vi "Command Information--SubVI.vi"(8 "error in (no error)":errorcluster, 9 "Instance":i32=1, 10 "Commands":T1=enum."Temp Feedback", 11 "Watlow F4T In":refnum<class "Watlow F4T.lvclass">) -> (0 "error out":errorcluster, 1 "Found?":bool, 2 "Register":T2, 3 "Watlow F4T Out":refnum<class "Watlow F4T.lvclass">)   [LabVIEW 2024, in "Watlow F4T.lvclass"]
uses:
  Watlow F4T.lvclass
  Controls/Standard Bus Register LUT Data--Cluster.ctl
  Controls/Standard Bus Commands--Enum.ctl
  Controls/Standard Bus Class Names--Enum.ctl
  Controls/Standard Bus Parameter Names--Enum.ctl
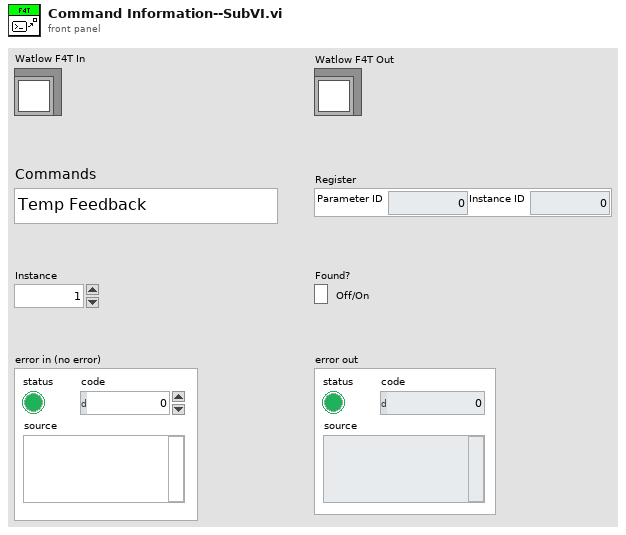
[diagram p1: front panel]
types:
  T1 = typedef "Watlow F4T.lvclass/Standard Bus Commands--Enum.ctl" = enum16{"Remote Setpoint", "Remote Mode", "Temp Feedback", "Target Setpoint", "Current Setpoint", "Setpoint Lower Limit", "Setpoint Upper Limit", "Ramp Rate Y", "Ramp Rate X", "Ramp Rate Action", "Temp Control State", "Temp Control Mode", "Power", "Heat Power", "Cool Power"}
  T2 = typedef "Watlow F4T.lvclass/Standard Bus Register LUT Data--Cluster.ctl" = cluster{"Parameter ID":i32, "Instance ID":i32}
  T3 = typedef "Watlow F4T.lvclass/Standard Bus Parameter Names--Enum.ctl" = enum16{"", "AC Line Frequency", "Actual IP Addressing Mode", "Actual Set Point", "Alarm Clearable", "Alarm Latched", "Alarm Silenced", "Alarm Source", "Alarm Source Instance", "Alarm Source Zone", "Alarm State", "Alarm Working Process Value", "Altitude Units", "Ambient Offset", "Ambient Temperature", "Analog", "Analog Input Value", "Analog Output Control Operation", "Analog Output Electrical Value", "Auto Transfer Type", "Auto-to-Manual Power", "Autotune", "Autotune Aggressiveness", "Autotune Set Point", "Autotune Status", "Available Logging Memory (MB)", "Available Logging Time (Hours)", "Barometric Pressure", "Baud Rate", "Blocking", "Calendar Start Day", "Calendar Start Hour", "Calendar Start Minute", "Calibration Offset", "Calibration Slope", "Cascade Control Mode Is Off", "Cascade Cool Power", "Cascade Heat Power", "Cascade Power", "Class", "Clear Active Level", "Clear Alarm", "Clear Error", "Clear Limit", "Closed-Loop Set Point", "Coefficient A", "Coefficient B", "Coefficient C", "Control Action", "Control Loop Control Mode Is Off", "Control Loop Error", "Control Loop Output Power", "Control Mode", "Control Mode Active", "Cool Algorithm", "Cool Output Curve", "Cool Power", "Cool Proportional Band 1", "Cool Proportional Band 2", "Cool Proportional Band 3", "Cool Proportional Band 4", "Cool Proportional Band 5", "Cool Proportional Band Inner Loop 1", "Cool Proportional Band Inner Loop 2", "Cool Proportional Band Inner Loop 3", "Cool Proportional Band Inner Loop 4", "Cool Proportional Band Inner Loop 5", "Cool Proportional Band Outer Loop 1", "Cool Proportional Band Outer Loop 2", "Cool Proportional Band Outer Loop 3", "Cool Proportional Band Outer Loop 4", "Cool Proportional Band Outer Loop 5", "Count", "Count Active Level", "Crossover Band", "Crossover Point", "Current Actual Power", "Current Error", "Current Gain", "Current Input Error Status", "Current Profile", "Current Read", "Current Step", "Data Map", "Data Type", "Date ", "Date Format", "Date of Manufacture", "Dead Band", "Delay Time", "Derivative 1", "Derivative 2", "Derivative 3", "Derivative 4", "Derivative 5", "Derivative Inner Loop 1", "Derivative Inner Loop 2", "Derivative Inner Loop 3", "Derivative Inner Loop 4", "Derivative Inner Loop 5", "Derivative Outer Loop 1", "Derivative Outer Loop 2", "Derivative Outer Loop 3", "Derivative Outer Loop 4", "Derivative Outer Loop 5", "Detection Threshold", "Device Name", "Device Status", "Digital", "Direction", "Disable Active Level", "Display", "Display Precision", "Display Units", "Elapsed Time", "Electrical Input Offset", "Electrical Input Slope", "Electrical Measurement", "Electrical Output Offset", "Electrical Output Slope", "End Action Loop 1", "End Action Loop 2", "End Action Loop 3", "End Action Loop 4", "Error", "Error Handling", "EtherNet/IP Enable", "Event 1", "Event 2", "Event 3", "Event 4", "Event 5", "Event 6", "Event 7", "Event 8", "File Size Limit (MB)", "File Type", "Filter", "Filtered Process Value", "Firmware Branch Number", "Fixed IP Gateway Part 1", "Fixed IP Gateway Part 2", "Fixed IP Gateway Part 3", "Fixed IP Gateway Part 4", "Fixed IP Gateway Part 5", "Fixed IP Gateway Part 6", "Fixed Power", "Fixed Time Base", "Function", "Guaranteed Soak Deviation 1", "Guaranteed Soak Deviation 2", "Guaranteed Soak Deviation 3", "Guaranteed Soak Deviation 4", "Guaranteed Soak Enable 1", "Guaranteed Soak Enable 2", "Guaranteed Soak Enable 3", "Guaranteed Soak Enable 4", "Hardware ID", "Heat Algorithm", "Heat Power", "Heat Proportional Band 1", "Heat Proportional Band 2", "Heat Proportional Band 3", "Heat Proportional Band 4", "Heat Proportional Band 5", "Heat Proportional Band Inner Loop 1", "Heat Proportional Band Inner Loop 2", "Heat Proportional Band Inner Loop 3", "Heat Proportional Band Inner Loop 4", "Heat Proportional Band Inner Loop 5", "Heat Proportional Band Outer Loop 1", "Heat Proportional Band Outer Loop 2", "Heat Proportional Band Outer Loop 3", "Heat Proportional Band Outer Loop 4", "Heat Proportional Band Outer Loop 5", "Heater Error", "Heater Offset", "High Limit Set Point", "High Power Scale", "High Set Point", "Hours", "Hysteresis", "IP Actual Address Part 1", "IP Actual Address Part 2", "IP Actual Address Part 3", "IP Actual Address Part 4", "IP Actual Address Part 5", "IP Actual Address Part 6", "IP Address Mode", "IP Fixed Address Part 1", "IP Fixed Address Part 2", "IP Fixed Address Part 3", "IP Fixed Address Part 4", "IP Fixed Address Part 5", "IP Fixed Address Part 6", "IP Fixed Subnet Part 1", "IP Fixed Subnet Part 2", "IP Fixed Subnet Part 3", "IP Fixed Subnet Part 4", "IP Fixed Subnet Part 5", "IP Fixed Subnet Part 6", "IP Version", "Idle Set Point", "Indicate Reading", "Inner Loop Cool Algorithm", "Inner Loop Deadband", "Inner Loop Heat Algorithm", "Inner Loop On/Off Cool Hysteresis", "Inner Loop On/Off Heat Hysteresis", "Inner Loop PID Set Active", "Inner Loop Set Point Closed", "Input A Turn Off", "Input A Turn On", "Input B Turn Off", "Input B Turn On", "Input Error", "Input Error Latching", "Input Error Power", "Input Point 1", "Input Point 10", "Input Point 2", "Input Point 3", "Input Point 4", "Input Point 5", "Input Point 6", "Input Point 7", "Input Point 8", "Input Point 9", "Input Scaling", "Input State", "Input Type", "Integral 1", "Integral 2", "Integral 3", "Integral 4", "Integral 5", "Integral Inner Loop 1", "Integral Inner Loop 2", "Integral Inner Loop 3", "Integral Inner Loop 4", "Integral Inner Loop 5", "Integral Outer Loop 1", "Integral Outer Loop 2", "Integral Outer Loop 3", "Integral Outer Loop 4", "Integral Outer Loop 5", "Jump Count", "Jump Step", "Key Action", "Latching", "Limit State", "Limit Status", "Load Current RMS", "Load Value", "Log Action", "Log Data", "Log Enable", "Log Interval", "Log To", "Logging Status", "Logic", "Low Limit Set Point", "Low Power Scale", "Low Set Point", "MAC Address", "Manual Power", "Maximum Manual Power", "Maximum Set Point", "Measure CJC", "Member", "Memory Full Action", "Message", "Message Enable", "Minimum Manual Power", "Minimum Off Time", "Minimum On Time", "Minimum Set Point", "Minutes", "Modbus Address", "Modbus TCP Enable", "Modbus Word Order", "Monitored Output", "Month", "Name", "Non-Volatile Save", "Number of PID Sets", "Off Active Level", "Off Delay", "Offset", "On/Off Cool Hysteresis", "On/Off Heat Hysteresis", "Open Loop Detect Deviation", "Open Loop Detect Enable", "Open Loop Detect Time", "Open-Loop Working Power", "Outer Loop Cool Algorithm", "Outer Loop Deadband", "Outer Loop Heat Algorithm", "Outer Loop Set Point Closed", "Output", "Output 1 Size", "Output 2 Size", "Output 3 Size", "Output 4 Size", "Output Function Instance", "Output Order", "Output Point 1", "Output Point 10", "Output Point 2", "Output Point 3", "Output Point 4", "Output Point 5", "Output Point 6", "Output Point 7", "Output Point 8", "Output Point 9", "Output Power", "Output Source Zone", "Output State", "Output Type", "Output Value", "Output Value 1", "Output Value 2", "Output Value 3", "Output Value 4", "PID Set 1 to 2 Crossover", "PID Set 2 to 3 Crossover", "PID Set 3 to 4 Crossover", "PID Set 4 to 5 Crossover", "PID Set Active", "PID Set Crossover", "Parity", "Part Number", "Pause / Resume Active Level", "Peltier Delay", "Power Out Hours", "Power Out Minutes", "Pressure Units", "Process Error Enable", "Process Error Low Value", "Produced Set Point 1", "Produced Set Point 2", "Produced Set Point 3", "Produced Set Point 4", "Profile Action Request", "Profile End Action", "Profile Number", "Profile Paused", "Profile Running", "Profile State", "RTD Lead Resistance", "RTD Leads", "Ramp Action", "Ramp Rate", "Ramp Scale", "Range High", "Range Low", "Rate", "Remote Set Point", "Remote Set Point Type", "Remote Transfer Interval In Hours", "Remote Transfer on Percent full", "Reset Active Level", "Resistance Range", "Restore Settings From", "Run Active Level", "Running", "Scale High", "Scale Low", "Seconds", "Sensor Type", "Serial Number", "Set Point", "Sides", "Silence Active Level", "Silence Alarm", "Silencing", "Simple Set Point Enable", "Software Build Number", "Software ID", "Software Prototype Version", "Software Release Version", "Source Function A", "Source Function B", "Source Function C", "Source Function D", "Source Function E", "Source Function F", "Source Function G", "Source Function H", "Source Instance A", "Source Instance B", "Source Instance C", "Source Instance D", "Source Instance E", "Source Instance F", "Source Instance G", "Source Instance H", "Source Value A", "Source Value B", "Source Value C", "Source Value D", "Source Value E", "Source Value F", "Source Value G", "Source Value H", "Source Zone A", "Source Zone B", "Source Zone C", "Source Zone D", "Source Zone E", "Source Zone F", "Source Zone G", "Source Zone H", "Start / Stop Active Level", "Start Active Level", "Start Profile", "Start Step", "Status", "Step Time Remaining", "Step Type", "TC Linearization", "TRU-TUNE+ Band", "TRU-TUNE+ Enable", "TRU-TUNE+ Gain", "Target Set Point", "Target Set Point Loop 1", "Target Set Point Loop 2", "Target Set Point Loop 3", "Target Set Point Loop 4", "Target Value", "Terminate", "Thermistor Curve", "Time", "Time Base Type", "Time Delay", "Time Format", "Time of Day", "Tolerance", "Transfer Files Now by", "Transmitter Active Level", "Type", "Units", "Unknown", "Value", "Valve Travel Time", "Wait For Process 1 Condition", "Wait For Process 1 Value", "Wait For Process 2 Condition", "Wait For Process 2 Value", "Wait For Process 3 Condition", "Wait For Process 3 Value", "Wait For Process 4 Condition", "Wait For Process 4 Value", "Year"}
  T4 = typedef "Watlow F4T.lvclass/Standard Bus Class Names--Enum.ctl" = enum16{"Alarm", "Analog Output", "Assembly", "Assembly Setup", "Cascade", "Compare", "Control Loop", "Counter", "Current", "Data Logging", "Device", "Digital I/O", "Digital Input", "Digital Output Fast", "Digital Output Limit", "Digital Output Slow", "Display", "Ethernet", "Function", "Function Key", "Limit", "Linearization", "Logging Point", "Logic", "Math", "Message", "Modbus", "Process Value", "Profile", "Real Time Clock", "Temperature Input", "Thermistor Input", "Timer", "Universal Input", "Variable"}
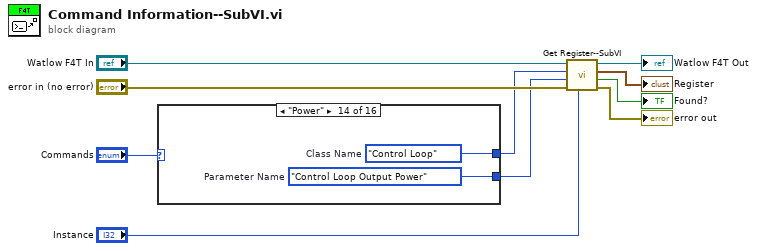
[diagram p0: block diagram]
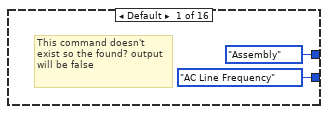
[diagram p2: hidden frame]
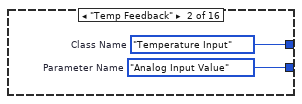
[diagram p3: hidden frame]
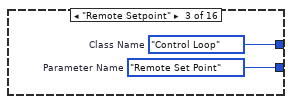
[diagram p4: hidden frame]
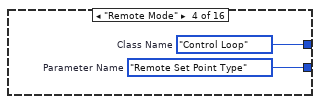
[diagram p5: hidden frame]
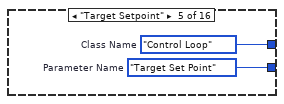
[diagram p6: hidden frame]
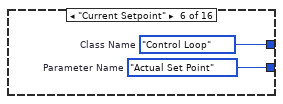
[diagram p7: hidden frame]
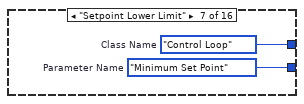
[diagram p8: hidden frame]
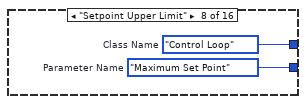
[diagram p9: hidden frame]
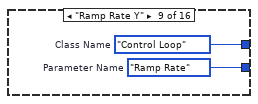
[diagram p10: hidden frame]
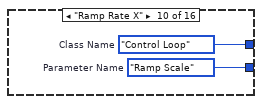
[diagram p11: hidden frame]
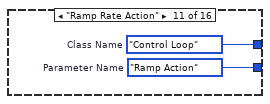
[diagram p12: hidden frame]
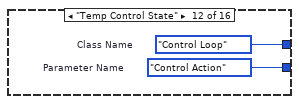
[diagram p13: hidden frame]
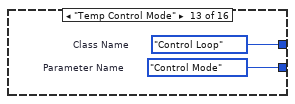
[diagram p14: hidden frame]
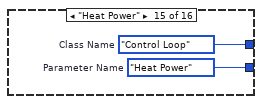
[diagram p15: hidden frame]
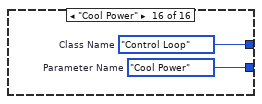
[diagram p16: hidden frame]
diagram:
  n1 = case shown="\"Power\"" "Commands" {
    tunnel: [Standard_Bus_Parameter_Names--Enum."AC Line Frequency" ("Parameter Name") w14 w16 w18 w20 w22 w24 w26 w28 w30 w32 w34 w36 w38 w40 w42] -> w8
    tunnel: [Standard_Bus_Class_Names--Enum."Assembly" ("Class Name") w13 w15 w17 w19 w21 w23 w25 w27 w29 w31 w33 w35 w37 w39 w41] -> w7
    frame Default {
      # "This command doesn't exist so the found? output will be false"
    }
    frame "Temp Feedback" {
      w14 = Standard_Bus_Parameter_Names--Enum."Analog Input Value"  # Parameter Name
      w13 = Standard_Bus_Class_Names--Enum."Temperature Input"  # Class Name
    }
    frame "Remote Setpoint" {
      w16 = Standard_Bus_Parameter_Names--Enum."Remote Set Point"  # Parameter Name
      w15 = Standard_Bus_Class_Names--Enum."Control Loop"  # Class Name
    }
    frame "Remote Mode" {
      w18 = Standard_Bus_Parameter_Names--Enum."Remote Set Point Type"  # Parameter Name
      w17 = Standard_Bus_Class_Names--Enum."Control Loop"  # Class Name
    }
    frame "Target Setpoint" {
      w20 = Standard_Bus_Parameter_Names--Enum."Target Set Point"  # Parameter Name
      w19 = Standard_Bus_Class_Names--Enum."Control Loop"  # Class Name
    }
    frame "Current Setpoint" {
      w22 = Standard_Bus_Parameter_Names--Enum."Actual Set Point"  # Parameter Name
      w21 = Standard_Bus_Class_Names--Enum."Control Loop"  # Class Name
    }
    frame "Setpoint Lower Limit" {
      w24 = Standard_Bus_Parameter_Names--Enum."Minimum Set Point"  # Parameter Name
      w23 = Standard_Bus_Class_Names--Enum."Control Loop"  # Class Name
    }
    frame "Setpoint Upper Limit" {
      w26 = Standard_Bus_Parameter_Names--Enum."Maximum Set Point"  # Parameter Name
      w25 = Standard_Bus_Class_Names--Enum."Control Loop"  # Class Name
    }
    frame "Ramp Rate Y" {
      w28 = Standard_Bus_Parameter_Names--Enum."Ramp Rate"  # Parameter Name
      w27 = Standard_Bus_Class_Names--Enum."Control Loop"  # Class Name
    }
    frame "Ramp Rate X" {
      w30 = Standard_Bus_Parameter_Names--Enum."Ramp Scale"  # Parameter Name
      w29 = Standard_Bus_Class_Names--Enum."Control Loop"  # Class Name
    }
    frame "Ramp Rate Action" {
      w32 = Standard_Bus_Parameter_Names--Enum."Ramp Action"  # Parameter Name
      w31 = Standard_Bus_Class_Names--Enum."Control Loop"  # Class Name
    }
    frame "Temp Control State" {
      w34 = Standard_Bus_Parameter_Names--Enum."Control Action"  # Parameter Name
      w33 = Standard_Bus_Class_Names--Enum."Control Loop"  # Class Name
    }
    frame "Temp Control Mode" {
      w36 = Standard_Bus_Parameter_Names--Enum."Control Mode"  # Parameter Name
      w35 = Standard_Bus_Class_Names--Enum."Control Loop"  # Class Name
    }
    frame "Power" {
      w38 = Standard_Bus_Parameter_Names--Enum."Control Loop Output Power"  # Parameter Name
      w37 = Standard_Bus_Class_Names--Enum."Control Loop"  # Class Name
    }
    frame "Heat Power" {
      w40 = Standard_Bus_Parameter_Names--Enum."Heat Power"  # Parameter Name
      w39 = Standard_Bus_Class_Names--Enum."Control Loop"  # Class Name
    }
    frame "Cool Power" {
      w42 = Standard_Bus_Parameter_Names--Enum."Cool Power"  # Parameter Name
      w41 = Standard_Bus_Class_Names--Enum."Control Loop"  # Class Name
    }
  }
  n2 = call "Get Register--SubVI.vi"("Instance"="Instance", "error in"="error in (no error)", "Parameter Name"=w8, "Class Name"=w7, "Watlow F4T in"="Watlow F4T In") -> ("error out"=→"error out":errorcluster, "Found?"=→"Found?":bool, "Register"=→"Register":T2, "Watlow F4T Out"=→"Watlow F4T Out":refnum<class "Watlow F4T.lvclass">)  [unwired: 3 in]
